vi "ConfWrite.vi"(8 "error in":errorcluster, 11 "StructIn":T1) -> (0 "error out":errorcluster, 3 "StructOut":T1)   [LabVIEW 2021, in "LibDan.lvlib"]
uses:
  LibDan.lvlib
  TerminalDef.ctl
  <vilib>/Utility/config.llb/Config Data RefNum.ctl
  <vilib>/Utility/config.llb/Write Key (String).vi
  <vilib>/Utility/config.llb/NI_LVConfig.lvlib
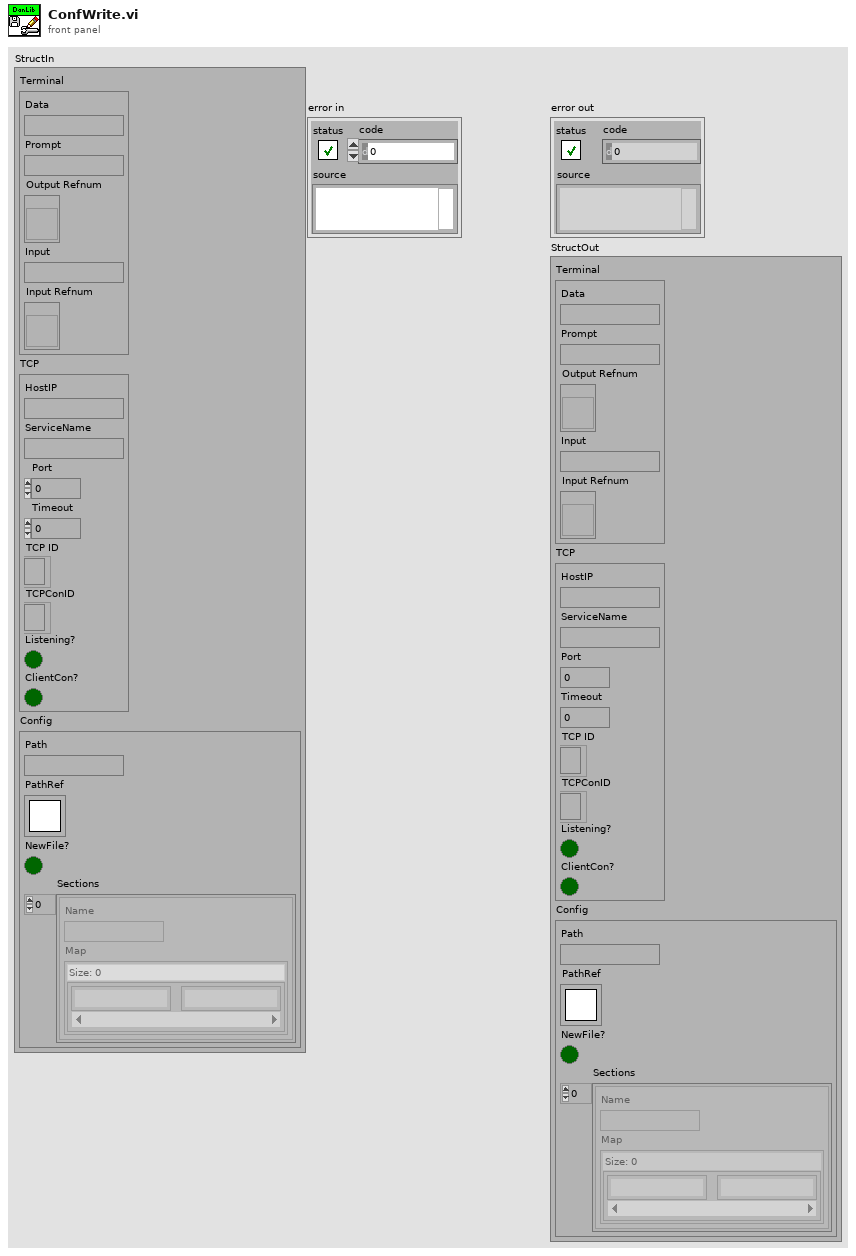
[diagram p1: front panel]
types:
  T1 = typedef "LibDan.lvlib/TerminalDef.ctl" = cluster{"Terminal":cluster{"Data":string, "Prompt":string, "Output Refnum":refnum<vi>, "Input":string, "Input Refnum":refnum<vi>}, "TCP":cluster{"HostIP":string, "ServiceName":string, "Port":u16, "Timeout":i32, "TCP ID":refnum<k5>, "TCPConID":refnum<k5>, "Listening?":bool, "ClientCon?":bool}, "Config":cluster{"Path":path, "PathRef":T2, "NewFile?":bool, "Sections":cluster{"Name":string, "Map":map{string, string}}[]}}
  T2 = typedef "NI_LVConfig.lvlib/Config Data RefNum.ctl" = refnum<k1>
  T3 = cluster{"Name":string, "Map":map{string, string}}[]
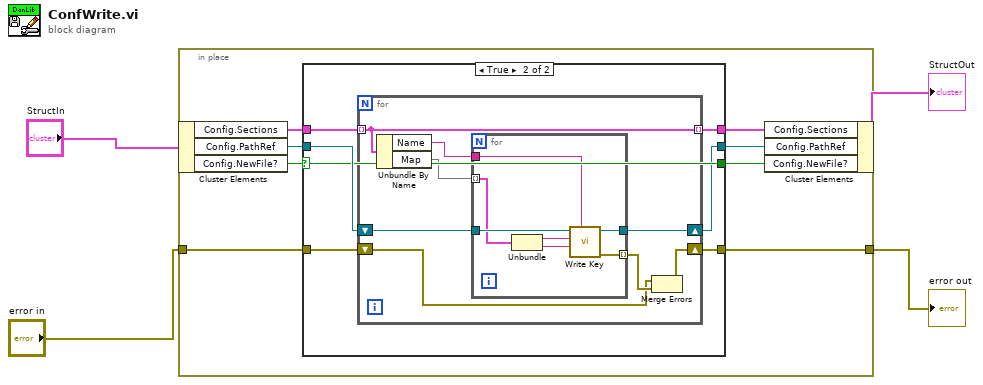
[diagram p0: block diagram]
diagram:
  n1 = in-place {
    in-place-border: "error in" -> [w7]
    in-place-border: [w6] -> w1
    n2 = in-place-cluster #1("StructIn") -> ("Config.Sections"=w9:T3, "Config.PathRef"=w11:T2, "Config.NewFile?"=w12:bool)
    n3 = case shown="True" w12 {
      selector: w12 -> [w15 w22]
      tunnel: w11 -> [w16 w23]
      tunnel: [w16 w17] -> w10
      tunnel: [w15 w22] -> w5
      tunnel: w9 -> [w14 w21]
      tunnel: [w14 w20] -> w8
      tunnel: w7 -> [w13 w19]
      tunnel: [w13 w18] -> w6
      frame False {
      }
      frame True {
        n4 = for {
          shift-right: [w30] -> w17
          shift-left: w23 -> [w31]
          tunnel: w21 -> [w28] mode=indexing
          tunnel: [w28] -> w20 mode=indexing
          shift-right: [w26] -> w18
          shift-left: w19 -> [w24]
          n5 = Unbundle By Name(w28) -> ("Name"=w29:string, "Map"=w27:map{string, string})
          n6 = for {
            tunnel: w31 -> [w38]
            tunnel: [w37] -> w30
            tunnel: w29 -> [w36]
            tunnel: w27 -> [w35] mode=indexing
            tunnel: [w32] -> w25 mode=indexing
            n7 = Unbundle(w35) -> (w34:string, w33:string)
            n8 = call-poly <vilib>:"Write Key.vi"("section"=w36, "value"=w33, "key"=w34, "refnum"=w38) -> ("error out"=w32:errorcluster, "refnum out"=w37:T2)  [unwired: 5 in, 1 out]
          }
          n9 = Merge Errors(w24, w25) -> (w26:errorcluster)
        }
      }
    }
    n10 = in-place-cluster #1("Config.Sections"=w8, "Config.PathRef"=w10, "Config.NewFile?"=w5) -> (→"StructOut":T1)
  }
  "error out" <- w1
